vi "SendText .vi"(4 "Body":string, 5 "Carrier":enum16{"T-Mobile", "AT&T", "Verizon", "Sprint"}(ring), 6 "Subject":string, 7 "phone number":string, 10 "Password":string, 11 "Email":string) -> ()   [LabVIEW 2018]
uses:
  <vilib>/smtpClient/Set Message Text.vi
  <vilib>/smtpClient/LabVIEWSMTPClient.lvlib
panel:
  in  "error in (no error)":errorcluster
  in  "TLS":bool=TRUE
  in  "Outgoing Mail Server (SMTP)":string="smtp.gmail.com"
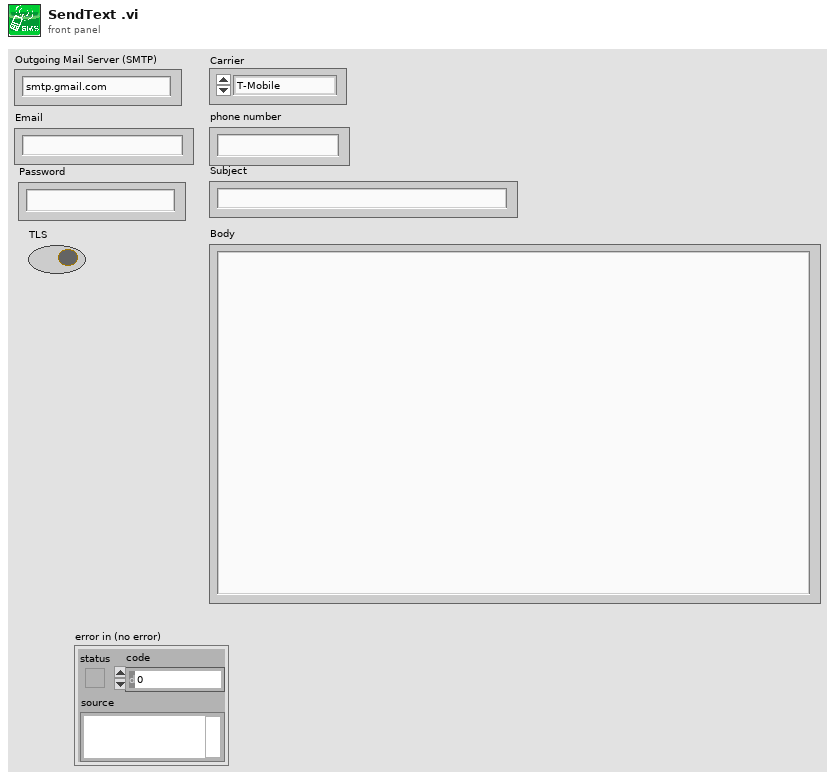
[diagram p1: front panel]
types:
  T1 = typedef "LabVIEWSMTPClient.lvlib/SmtpClientHandle.ctl" = refnum<k1>
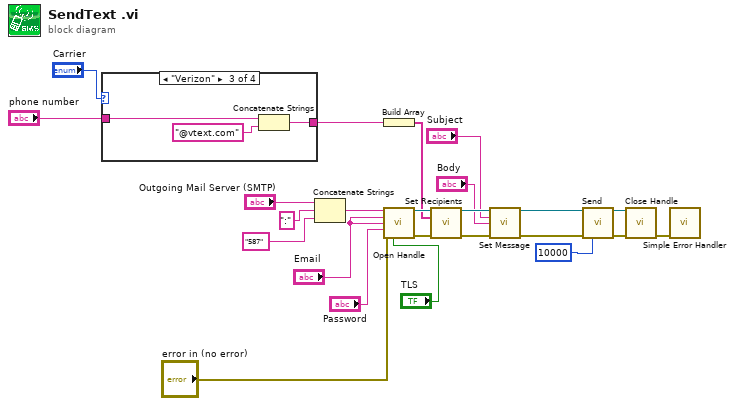
[diagram p0: block diagram]
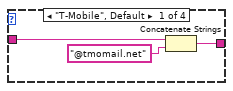
[diagram p2: hidden frame]
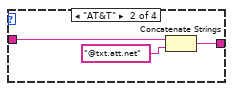
[diagram p3: hidden frame]
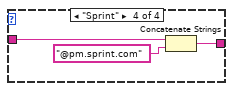
[diagram p4: hidden frame]
diagram:
  n1 = case shown="\"Verizon\"" "Carrier" {
    tunnel: "phone number" -> [w27 w29 w32 w35]
    tunnel: [w25 w30 w33 w36] -> w10
    frame "T-Mobile", Default {
      n2 = Concatenate Strings(w27, "@tmomail.net" ("string")) -> (w25:string)
    }
    frame "AT&T" {
      n3 = Concatenate Strings(w29, "@txt.att.net" ("string")) -> (w30:string)
    }
    frame "Verizon" {
      n4 = Concatenate Strings(w32, "@vtext.com" ("string")) -> (w33:string)
    }
    frame "Sprint" {
      n5 = Concatenate Strings(w35, "@pm.sprint.com") -> (w36:string)
    }
  }
  n6 = Concatenate Strings("Outgoing Mail Server (SMTP)", ":" ("string"), "587" ("Port")) -> (w5:string)
  n7 = Build Array(w10) -> (w9:string[])
  n8 = call <vilib>:"Open Handle.vi"("server address"=w5, "from"="Email", "username"="Email", "password"="Password", "error in (no error)"="error in (no error)", "use TLS (false)"="TLS") -> ("handle out"=w22:T1, "error out"=w19:errorcluster)  [unwired: 8 in]
  n9 = call <vilib>:"Set Recipients.vi"("handle in"=w22, "to"=w9, "error in (no error)"=w19) -> ("handle out"=w18:T1, "error out"=w17:errorcluster)  [unwired: 11 in]
  n10 = call-poly <vilib>:"Set Message.vi"("handle in"=w18, "subject"="Subject", "plain text message"="Body", "error in (no error)"=w17) -> ("handle out"=w14:T1, "error out"=w13:errorcluster)  [unwired: 10 in]
  n11 = call <vilib>:"Send.vi"("handle in"=w14, "error in (no error)"=w13, "timeout in ms (10000)"=10000) -> ("handle out"=w12:T1, "error out"=w11:errorcluster)  [unwired: 10 in, 1 out]
  n12 = call <vilib>:"Close Handle.vi"("handle in"=w12, "error in (no error)"=w11) -> ("error out"=w2:errorcluster)  [unwired: 12 in, 1 out]
  n13 = call <vilib>:"Simple Error Handler.vi"("error in (no error)"=w2) -> ()  [unwired: 4 in, 5 out]
